vi "SetConnectedStatus.vi"(6 "status":T1, 7 "dvrConnected":T2) -> (3 "dvrConnected":T2)   [LabVIEW 2017, in "ServerComm.lvlib"]
uses:
  <vilib>/addons/InsightCM/Devices/Shared/Common/ServerComm/ServerComm.lvlib
  <vilib>/addons/InsightCM/Devices/Shared/Common/ServerComm/controls/ConnectedStatusDvr.ctl
  <vilib>/addons/InsightCM/Devices/Shared/Common/ServerComm/controls/ConnectionStatus.ctl
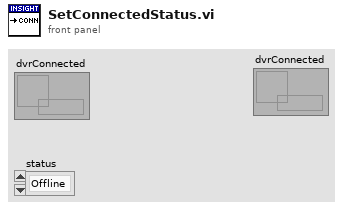
[diagram p1: front panel]
types:
  T1 = typedef "ServerComm.lvlib/ConnectionStatus.ctl" = enum16{"Offline", "NotAuthorized", "Online"}
  T2 = typedef "ServerComm.lvlib/ConnectedStatusDvr.ctl" = refnum<data-value>
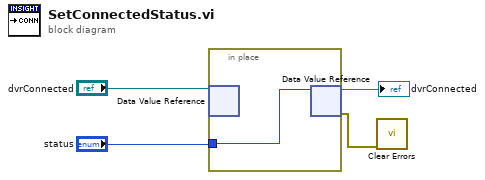
[diagram p0: block diagram]
diagram:
  n1 = in-place {
    in-place-border: "status" -> [w5]
    n2 = in-place-dvr #1("dvrConnected") -> ()  [unwired: 2 out]
    n3 = in-place-dvr #1(w5) -> (→"dvrConnected":T2, w2:errorcluster)
  }
  n4 = call <vilib>:"Clear Errors.vi"("error in (no error)"=w2) -> ()  [unwired: 5 in, 2 out]
